vi "DtCreateAinChan.vi"(1 "Channel Type":i32(ring)=100 items=["SingleEnded"=100, "Differential"=101], 2 "Range Min":dbl=-10.0, 3 "Range Max":dbl=10.0, 5 "Board Name":string, 7 "Channel":string="0", 9 "Element":u32, 11 "error in (no error)":errorcluster) -> (4 "Task out":i32, 8 "Actual Number of Channels":u32, 15 "error out":errorcluster)   [LabVIEW 2016]
doc: "Creates one or more virtual analog input channels to measure voltage.\n\nNote: If your device supports streaming digital inputs, counter/timers, and/or quadrature decoder inputs through the analog input subsystem, you must use the Analog Input - Raw instance of this VI to create virtual channels for the digital input ports, counter/timer channels, and/or quadrature decoder channels.\n\nLV-Link automatically configures the appropriate data encoding (binary or twos complement) and resolution for the subsystem, and sets the gain for all analog input channels to 1. To change the gain for individual channels, use the DtOLSetChanGain VI.\n\nTo read the value of one or more virtual analog input channels, use the DtOLRead VI."
uses:
  <userlib>/LV-Link3/DtLvLink.lvlib
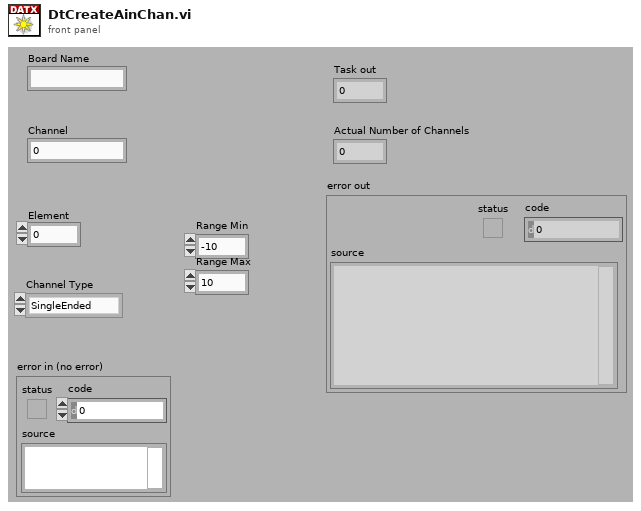
[diagram p1: front panel]
types:
  T1 = enum32{"AnalogInput", "AnalogOutput", "DigitalInput", "DigitalOutput", "Quadrature", "CounterTimer"}
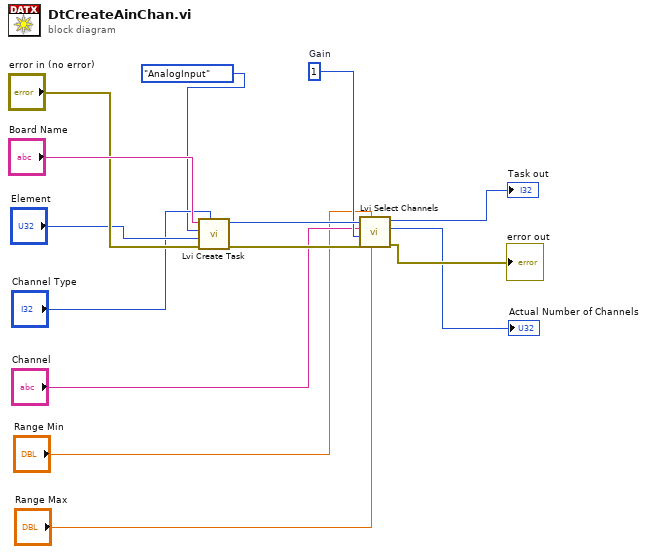
[diagram p0: block diagram]
diagram:
  w12 = u32 1  # Gain
  n1 = call <userlib>:"Lvi Create Task.vi"("SEorDiff"="Channel Type", "error in (no error)"="error in (no error)", "SubSysIndex"="Element", "ChanType"=T1."AnalogInput", "BoardName"="Board Name") -> ("error out"=w13:errorcluster, "TaskRef"=w14:i32)  [unwired: 4 in, 1 out]
  n2 = call <userlib>:"Lvi Select Channels.vi"("MaxRange"="Range Max", "MinRange"="Range Min", "error in (no error)"=w13, "Gain"=w12, "ChanListStr"="Channel", "TaskRef"=w14) -> ("error out"=→"error out":errorcluster, "ActualNumChannels"=→"Actual Number of Channels":u32, "TaskRef out"=→"Task out":i32)  [unwired: 2 in, 1 out]
